vi "PSTR-Update Frequency Ring.vi"(0 "Data":T1, 7 "Freq Ring":refnum<vi>) -> ()   [LabVIEW 2020]
uses:
  Typedefs/PSTR-Data.ctl
  Typedefs/PSTR-Model Fit.ctl
  Typedefs/PSTR-Fit Parameters.ctl
panel:
  # "NF x NL x 2 x Npts"
  # "NF x NL x Npts"
  # "NF x NL"
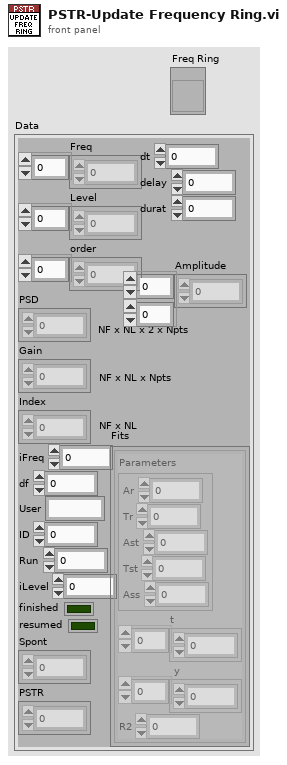
[diagram p1: front panel]
types:
  T1 = typedef "PSTR-Data.ctl" = cluster{"Freq":dbl[], "Level":dbl[], "order":i32[], "PSD":dbl[][][][], "Gain":dbl[][][], "Index":dbl[][], "iFreq":i32, "df":dbl, "User":string, "ID":i32, "Run":i32, "iLevel":i32, "finished":bool, "resumed":bool, "Spont":dbl[][], "PSTR":dbl[][][], "dt":dbl, "delay":dbl, "durat":dbl, "Fits":T2[][], "Amplitude":dbl[][]}
  T2 = typedef "PSTR-Model Fit.ctl" = cluster{"Parameters":T3, "t":dbl[], "y":dbl[], "R2":dbl}
  T3 = typedef "PSTR-Fit Parameters.ctl" = cluster{"Ar":dbl, "Tr":dbl, "Ast":dbl, "Tst":dbl, "Ass":dbl}
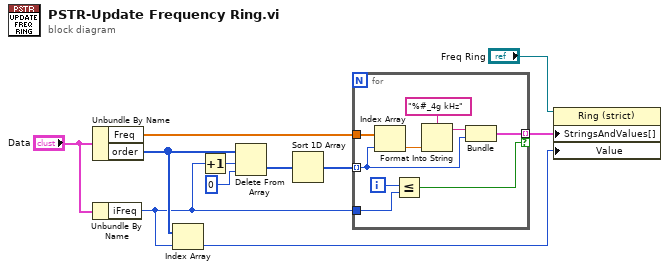
[diagram p0: block diagram]
diagram:
  n1 = Unbundle By Name("Data") -> ("Freq"=w10:dbl[], "order"=w5:i32[])
  n2 = Unbundle By Name("Data") -> ("iFreq"=w4:i32)
  n3 = Index Array(array=w5, index=w4) -> (element=w3:i32)
  n4 = Increment(x=w4) -> (x+1=w2:i32)
  n5 = Delete From Array(array=w5, length=w2, index=0) -> (deleted portion=w9:i32[])  [unwired: 1 out]
  n6 = Sort 1D Array(array=w9) -> (sorted array=w8:i32[])
  n7 = for {
    tunnel: w8 -> [w15] mode=indexing
    tunnel: [w12] -> w7 mode=indexing if=w17
    tunnel: w4 -> [w18]
    tunnel: w10 -> [w14]
    i -> [w19]
    n8 = Index Array(array=w14, index=w15) -> (element=w13:dbl)
    n9 = Less Or Equal?(x=w19, y=w18) -> (x <= y?=w17:bool)
    n10 = Format Into String(format string="%#_4g kHz", w13) -> (resulting string=w16:string)  [unwired: 2 in, 1 out]
    n11 = Bundle(w16, "Freq"=w15) -> (w12:cluster{string, "Freq":i32})  [unwired: 1 in]
  }
  n12 = property class="Ring (strict)"(reference="Freq Ring", "StringsAndValues[]"=w7, "Value"=w3) -> ()  [unwired: 1 in, 2 out]
